vi "Computing Resource Monitor.vi"(8 "error in (no error)":errorcluster) -> (0 "error out":errorcluster)   [LabVIEW 2023]
doc: "This VI uses the sys exec VI to pull computing resource usage stats and then parses the data into logical clusters for reading."
uses:
  <vilib>/Platform/TimedLoop/XDataNode/timing_clust.ctl
  <vilib>/Platform/TimedLoop/XDataNode/nitl_modes.ctl
  <vilib>/Platform/TimedLoop/XDataNode/wakeup.ctl
  <vilib>/platform/TimedLoop/XDataNode/XDataNode.xnode
  <vilib>/Platform/TimedLoop/XDataNode/XDNodeRunTimeDep.lvlib
panel:
  out "Linux Standard Out":string
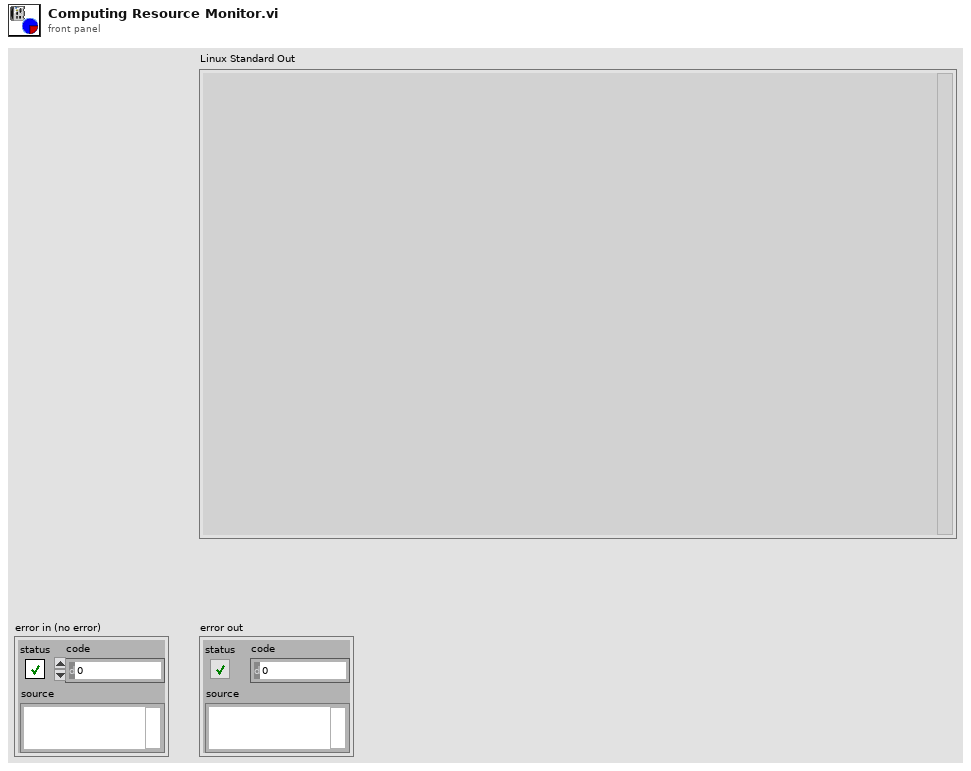
[diagram p1: front panel]
types:
  T1 = typedef "XDNodeRunTimeDep.lvlib/timing_clust.ctl" = cluster{"Expected End [f-1]":u64, "Actual End [f-1]":u64, "Finished Late? [f-1]":bool, "Expected End [i-1]":u64, "Actual End [i-1]":u64, "Finished Late? [i-1]":bool, "Expected Start [i]":u64, "Actual Start [i]":u64, "Expected Start [f]":u64, "Actual Start [f]":u64, "Source Name":string, "Structure Name":string, "Period":i64, "Deadline":i64, "Offset":i64, "Start":i64, "Priority":i32, "Timeout":i32, "Mode":T2, "Wakeup Reason":T3, "Error":errorcluster, "Source Type":string, "Secondary Source Type":string, "Global End Time":u64, "Global Start Time":u64, "Frame Duration":u64, "Iteration Duration":u64, "Assigned CPU":i32, "I/O Scan Engine Mode":u32}
  T2 = typedef "XDNodeRunTimeDep.lvlib/nitl_modes.ctl" = enum32{"No Change", "Process missed periods, maintain original phase", "Discard missed periods, maintain original phase", "Process missed periods, ignore original phase", "Discard missed periods, ignore original phase"}
  T3 = typedef "XDNodeRunTimeDep.lvlib/wakeup.ctl" = enum32{"Normal", "Aborted", "Asynchronous wakeup", "Timing source error", "Timed loop error", "Timeout"}
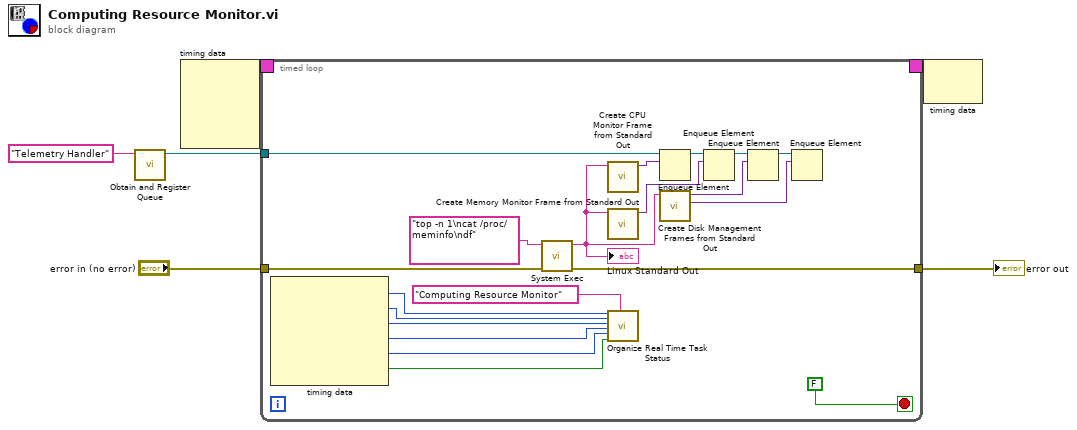
[diagram p0: block diagram]
diagram:
  n1 = call "Obtain and Register Queue.vi"("Queue Name (unnamed)"="Telemetry Handler" ("name (unnamed)")) -> ("Queue Reference"=w4:refnum<queue>)  [unwired: 9 in, 1 out]
  n2 = node-c288() -> (w6:T1)  [unwired: 4 in]
  n3 = timed-loop {
    tunnel: "error in (no error)" -> [w13]
    tunnel: [w25] -> w2
    tunnel: w4 -> [w23]
    timing: w6 -> [_]
    timing-out: [_] -> w5
    stop <- FALSE stop-if-true
    n4 = node-c288() -> (w19:i32, w18:i32, w17:i64, w16:i64, w15:i64, w14:bool)  [unwired: 1 in]
    n5 = call <vilib>:"System Exec.vi"("error in (no error)"=w13, "command line"="top -n 1\ncat /proc/meminfo\ndf") -> ("error out"=w25:errorcluster, "standard output"=w11:string)  [unwired: 6 in, 2 out]
    "Linux Standard Out" <- w11
    n6 = call "Create CPU Monitor Frame from Standard Out.vi"("Standard Output"=w11) -> ("Frame"=w24:variant)  [unwired: 10 in]
    n7 = call "Create Memory Monitor Frame from Standard Out.vi"("Starndard Output"=w11) -> ("Frame"=w21:variant)  [unwired: 10 in]
    n8 = call "Organize Real Time Task Status.vi"("Priority"=w19, "Processor"=w18, "Offset"=w17, "Iteration Duration"=w16, "Period"=w15, "Finished Late? [i-1]"=w14, "Task Name"="Computing Resource Monitor") -> ()  [unwired: 12 in, 1 out]
    n9 = Enqueue Element(queue=w23, element=w24) -> (queue out=w22:refnum<queue>)  [unwired: 2 in, 2 out]
    n10 = call "Create Disk Management Frames from Standard Out.vi"("Standard Output"=w11) -> ("Writeable Drives Frame"=w8:variant, "Disk Management Frame"=w9:variant)  [unwired: 9 in]
    n11 = Enqueue Element(queue=w22, element=w21) -> (queue out=w10:refnum<queue>)  [unwired: 2 in, 2 out]
    n12 = Enqueue Element(queue=w10, element=w9) -> (queue out=w7:refnum<queue>)  [unwired: 2 in, 2 out]
    n13 = Enqueue Element(queue=w7, element=w8) -> ()  [unwired: 2 in, 3 out]
  }
  "error out" <- w2
  n14 = node-c288(w5) -> ()  [unwired: 1 out]
